vi "PI VISA Receive Characters.vi"(0 "System no.":i32=1 min=1 step=1, 2 "Bytes to read":u16=1, 5 "error in":errorcluster) -> (14 "String read":string, 15 "Bytes read":u16, 19 "error out":errorcluster)   [LabVIEW 2026]
doc: "This VI reads n bytes (characters) via the chosen VISA interface. Sub-vi for PI Receive String.vi."
uses:
  Global1.vi
panel:
  out "VISA resource name":refnum<visa-resource-name>
  # "This vi reads n bytes (characters) via the chosen VISA interface."
  # "Communication setup indicators (for troubleshooting):"
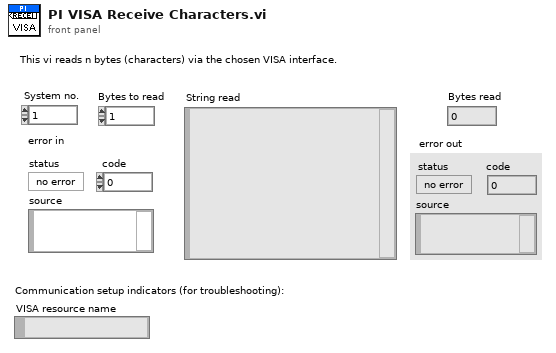
[diagram p1: front panel]
types:
  T1 = typedef "Available interfaces.ctl" = u16
  T2 = cluster{"RS232 Portnumber":i32, "Timeout":i32, "RS232 Baud rate":u32, "Interface":T1, "GPIB Bus":i32, "GPIB Address":i32, "GPIB Mode":i32}[]
  T3 = cluster{"RS232 Portnumber":i32, "Timeout":i32, "RS232 Baud rate":u32, "Interface":T1, "GPIB Bus":i32, "GPIB Address":i32, "GPIB Mode":i32}
  T4 = cluster{"Host address/name":string, "Port":i32, "Board":i32}[]
  T5 = cluster{"Host address/name":string, "Port":i32, "Board":i32}
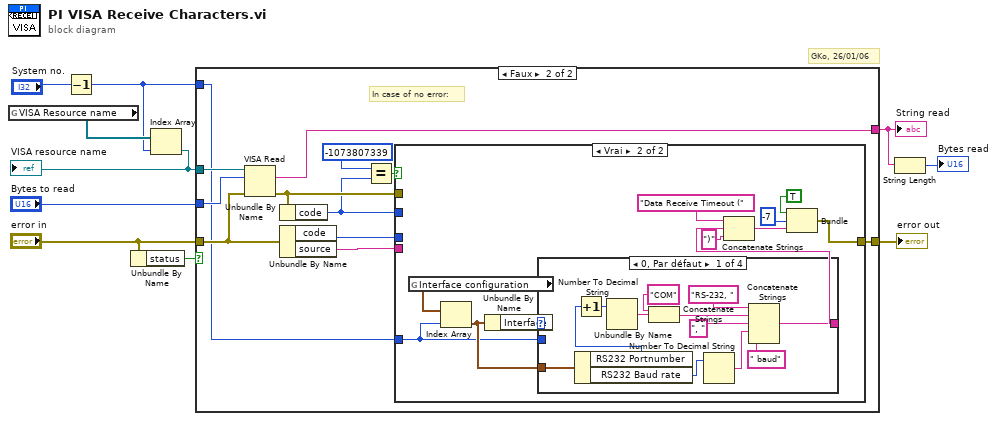
[diagram p0: block diagram]
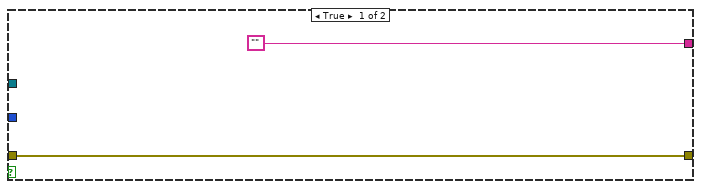
[diagram p2: hidden frame]
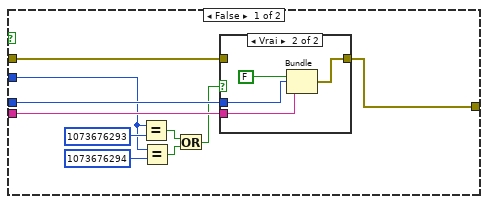
[diagram p3: hidden frame]
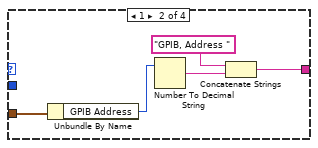
[diagram p5: hidden frame]
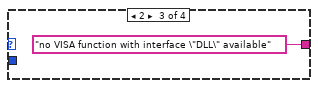
[diagram p6: hidden frame]
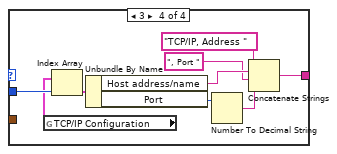
[diagram p7: hidden frame]
diagram:
  # "GKo, 26/01/06"
  n1 = global read "Global1.vi" "VISA Resource name"() -> (w3:refnum<visa-resource-name>[])
  n2 = Decrement(x="System no.") -> (x-1=w1:i32)
  n3 = Unbundle By Name("error in") -> ("status"=w7:bool)
  n4 = Index Array(array=w3, index=w1) -> (element=w2:refnum<visa-resource-name>)
  "VISA resource name" <- w2
  n5 = case shown="Faux" w7 {
    tunnel: "error in" -> [w12 w18]
    tunnel: [w12 w21] -> w10
    tunnel: ["" w20] -> w9
    tunnel: "Bytes to read" -> [_ w19]
    tunnel: w2 -> [_ w22]
    tunnel: w1 -> [_ w15]
    frame True {
    }
    frame False {
      # "In case of no error:"
      n6 = VISA Read(VISA resource name=w22, byte count=w19, error in (no error)=w18) -> (read buffer=w20:string, error out=w24:errorcluster)  [unwired: 2 out]
      n7 = Unbundle By Name(w24) -> ("code"=w13:i32)
      n8 = Unbundle By Name(w18) -> ("code"=w17:i32, "source"=w16:string)
      n9 = Equal?(x=-1073807339 ("y"), y=w13) -> (x = y?=w23:bool)
      n10 = case shown="Vrai" w23 {
        tunnel: w13 -> [w28 _]
        tunnel: [w34 w50] -> w21
        tunnel: w24 -> [w33 _]
        tunnel: w17 -> [w32 _]
        tunnel: w16 -> [w31 _]
        tunnel: w15 -> [_ w40]
        frame False {
          n11 = Equal?(x=w28, y=1073676293) -> (x = y?=w25:bool)
          n12 = Equal?(x=w28, y=1073676294) -> (x = y?=w27:bool)
          n13 = Or(x=w25, y=w27) -> (x .or. y?=w26:bool)
          n14 = case shown="Vrai" w26 {
            tunnel: [w35 w39] -> w34
            tunnel: w33 -> [w35 _]
            tunnel: w32 -> [_ w37]
            tunnel: w31 -> [_ w36]
            frame False {
            }
            frame True {
              n15 = Bundle(FALSE, "code"=w37, "source"=w36) -> (w39:cluster{bool, "code":i32, "source":string})  [unwired: 1 out]
            }
          }
        }
        frame True {
          n16 = global read "Global1.vi" "Interface configuration"() -> (w47:T2)
          n17 = Index Array(array=w47, index=w40) -> (element=w43:T3)
          n18 = Unbundle By Name(w43) -> ("Interface"=w44:T1)
          n19 = case shown="0, Par défaut" w44 {
            tunnel: w43 -> [w62 w66 _ _]
            tunnel: [w60 w63 "no VISA function with interface \"DLL\" available" ("string") w76] -> w42
            tunnel: w40 -> [_ _ _ w75]
            frame 0, Default {
              n20 = Unbundle By Name(w62) -> ("RS232 Portnumber"=w52:i32, "RS232 Baud rate"=w58:u32)
              n21 = Increment(x=w52) -> (x+1=w53:i32)
              n22 = Number To Decimal String(number=w53) -> (decimal integer string=w54:string)  [unwired: 1 out]
              n23 = Concatenate Strings("COM" ("string"), w54) -> (w51:string)
              n24 = Number To Decimal String(number=w58) -> (decimal integer string=w57:string)  [unwired: 1 out]
              n25 = Concatenate Strings("RS-232, " ("string"), w51, ", " ("string"), w57, " baud" ("string")) -> (w60:string)
            }
            frame 1 {
              n26 = Unbundle By Name(w66) -> ("GPIB Address"=w64:i32)
              n27 = Number To Decimal String(number=w64) -> (decimal integer string=w65:string)  [unwired: 1 out]
              n28 = Concatenate Strings("GPIB, Address " ("string"), w65) -> (w63:string)
            }
            frame 2 {
            }
            frame 3 {
              n29 = global read "Global1.vi" "TCP/IP Configuration"() -> (w74:T4)
              n30 = Index Array(array=w74, index=w75) -> (element=w73:T5)
              n31 = Unbundle By Name(w73) -> ("Host address/name"=w72:string, "Port"=w70:i32)
              n32 = Number To Decimal String(number=w70) -> (decimal integer string=w69:string)  [unwired: 1 out]
              n33 = Concatenate Strings("TCP/IP, Address " ("string"), w72, ", Port " ("string"), w69) -> (w76:string)
            }
          }
          n34 = Concatenate Strings("Data Receive Timeout (", w42, ")" ("string")) -> (w41:string)
          n35 = Bundle(TRUE, "count"=-7, w41) -> (w50:cluster{bool, "count":i32, string})  [unwired: 1 out]
        }
      }
    }
  }
  "error out" <- w10
  "String read" <- w9
  n36 = String Length(string=w9) -> (length=→"Bytes read":i32)
